vi "Remove Value.vi"(8 "error in (no error)":errorcluster, 10 "key":string, 11 "JSON Value in":refnum<class "JSON Value.lvclass">) -> (0 "error out":errorcluster, 2 "found":bool, 3 "JSON Value out":refnum<class "JSON Value.lvclass">)   [LabVIEW 2016, in "JSON Value.lvclass"]
doc: "Remove the given parameter from the specified JSON Object"
uses:
  JSON Value.lvclass
  JSON Value.lvclass/JSON Value.ctl
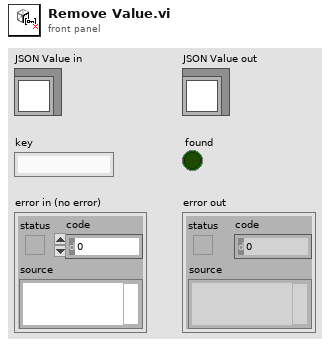
[diagram p1: front panel]
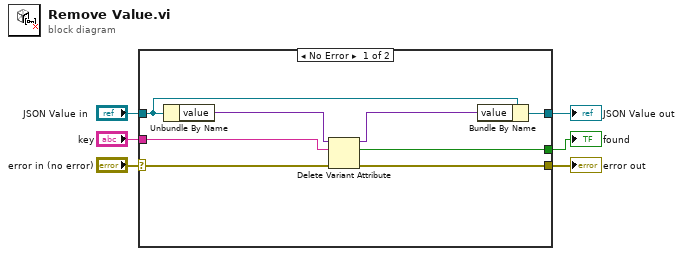
[diagram p0: block diagram]
diagram:
  n1 = case shown="No Error" "error in (no error)" {
    selector: "error in (no error)" -> [w13 w16]
    tunnel: [w11 w16] -> w5
    tunnel: "JSON Value in" -> [w9 w15]
    tunnel: "key" -> [w14 _]
    tunnel: [w10 _] -> w2
    tunnel: [w7 w15] -> w1
    frame No Error {
      n2 = Unbundle By Name(w9) -> ("value"=w12:variant)
      n3 = Delete Variant Attribute(4:w13, 6:w14, 7:w12) -> (0:w11:errorcluster, 2:w10:bool, 3:w8:variant)
      n4 = Bundle By Name(cluster=w9, "value"=w8) -> (w7:refnum<class "JSON Value.lvclass">)
    }
    frame Error {
    }
  }
  "error out" <- w5
  "found" <- w2
  "JSON Value out" <- w1
